vi "Current State.vi"(8 "error in (no error)":errorcluster, 10 "Elevator State":T1 {"Current Elevation" scale=0.0..100.0; "Current Travel Rate" scale=-1.0..1.0}, 11 "Elevator in":refnum<class "Elevator.lvclass">) -> (0 "error out":errorcluster, 3 "Elevator out":refnum<class "Elevator.lvclass">)   [LabVIEW 2014, in "Elevator.lvlib" / "Elevator.lvclass"]
uses:
  Elevator.lvclass
  Elevator State.ctl
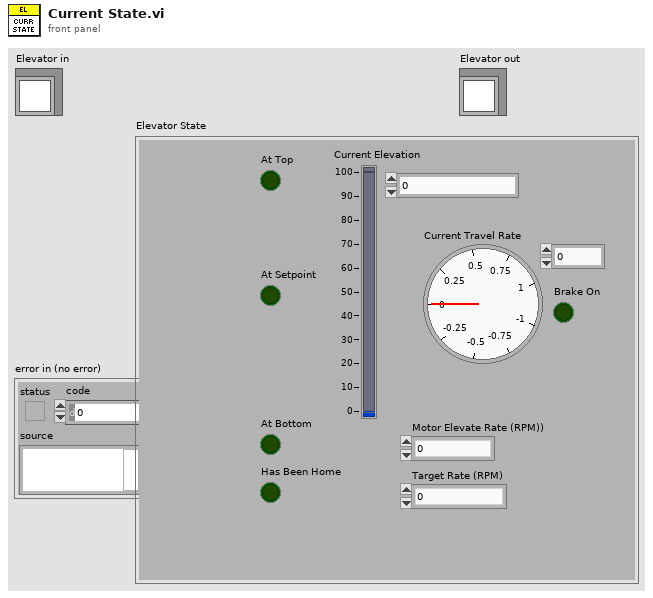
[diagram p1: front panel]
types:
  T1 = typedef "Elevator.lvlib/Elevator.lvclass/Elevator State.ctl" = cluster{"At Bottom":bool, "At Top":bool, "At Setpoint":bool, "Target Rate (RPM)":dbl, "Current Travel Rate":dbl, "Current Elevation":dbl, "Brake On":bool, "Motor Elevate Rate (RPM))":dbl, "Has Been Home":bool}
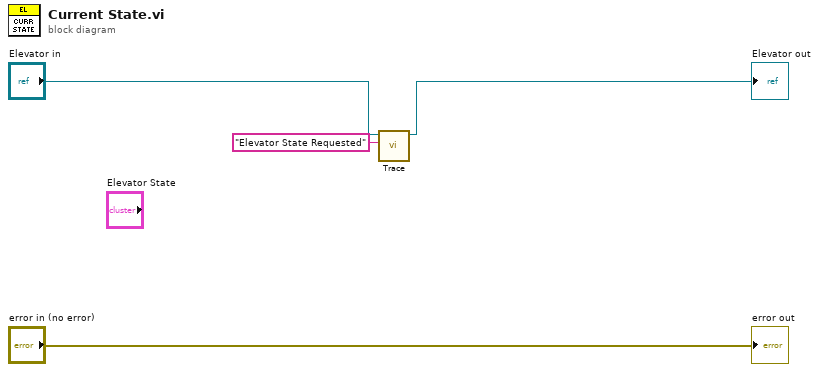
[diagram p0: block diagram]
diagram:
  n1 = call-dynamic "Trace.vi"("System Action"="Elevator State Requested", "System Actor in"="Elevator in") -> ("System Actor out"=→"Elevator out":refnum<class "Elevator.lvclass">)  [unwired: 8 in, 1 out]
  "error out" <- "error in (no error)"
